vi "ADV Results Initiate.vi"(8 "error in":errorcluster, 10 "DAC ADV.lvclass":refnum<class "DAC ADV.lvclass">, 11 "Water Tunnel Results in":refnum<class "Water Tunnel Results.lvclass">) -> (0 "error out":errorcluster, 3 "Water Tunnel Results out":refnum<class "Water Tunnel Results.lvclass">)   [LabVIEW 2019, in "Results.lvlib" / "Water Tunnel Results.lvclass"]
uses:
  Water Tunnel Results.lvclass
  Water Tunnel Results.lvclass/Water Tunnel Results.ctl
  DAC/Water Tunnel/ADV/DAC ADV.lvclass
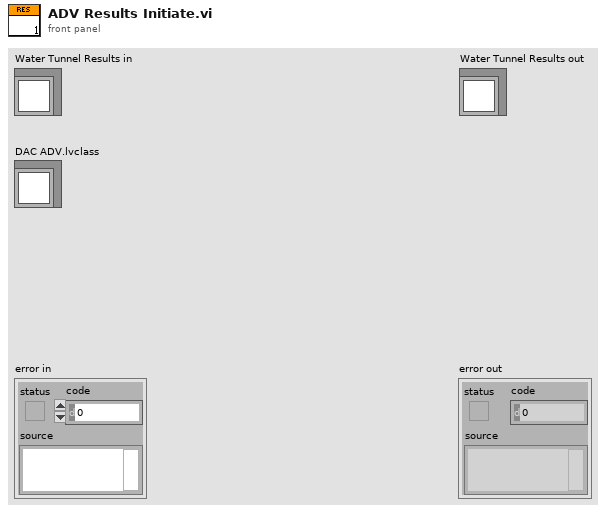
[diagram p1: front panel]
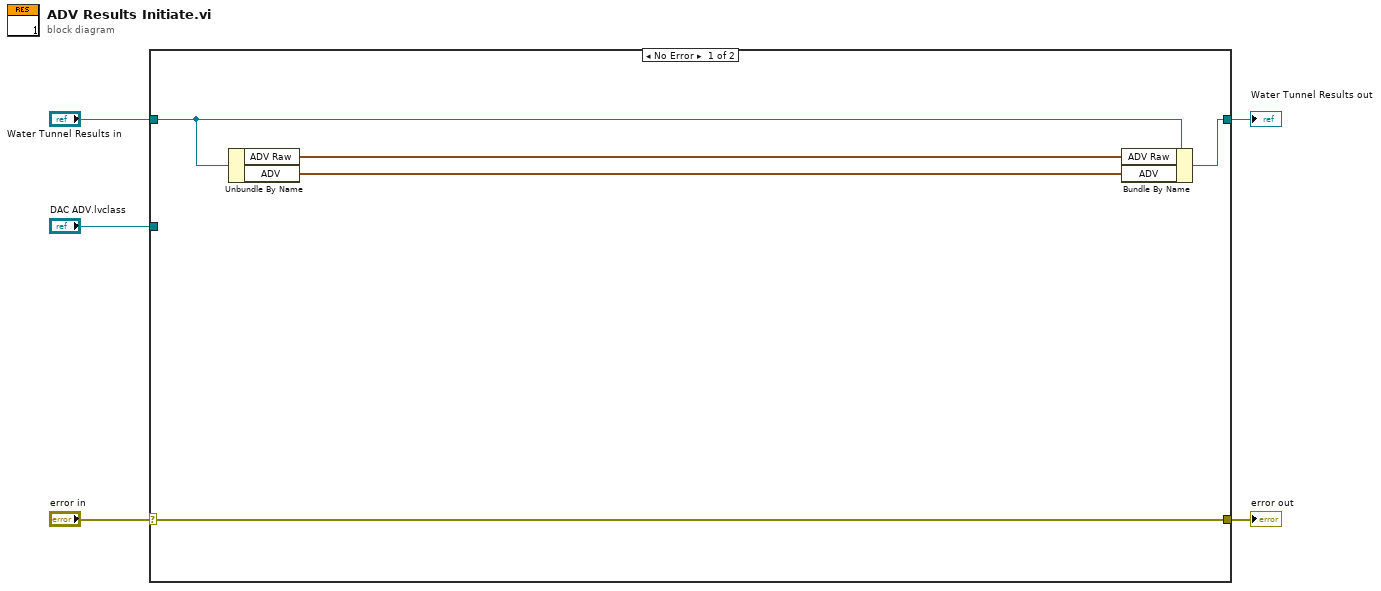
[diagram p0: block diagram]
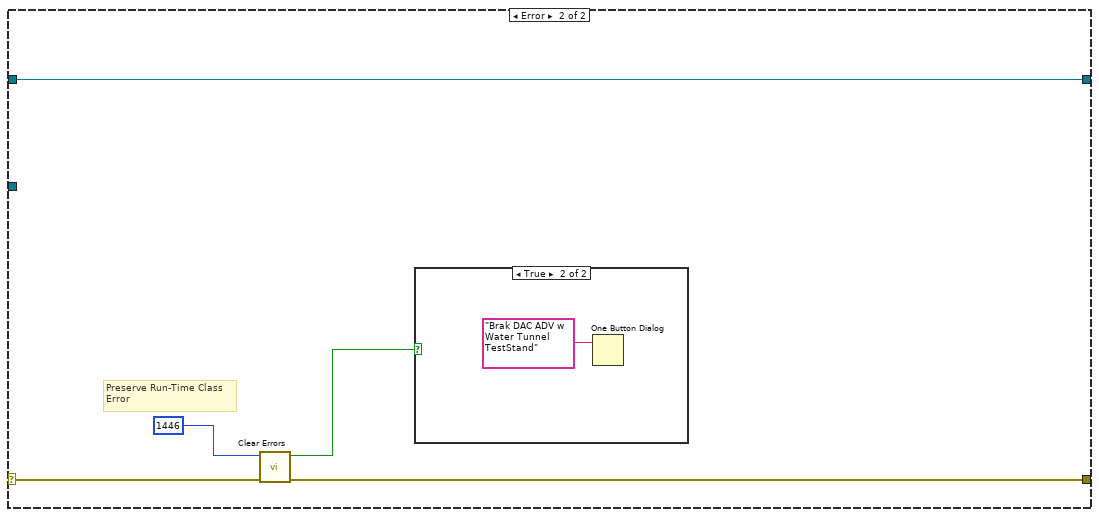
[diagram p2: hidden frame]
diagram:
  n1 = case shown="No Error" "error in" {
    selector: "error in" -> [w10 w14]
    tunnel: [w10 w13] -> w4
    tunnel: [w9 w15] -> w2
    tunnel: "Water Tunnel Results in" -> [w8 w15]
    tunnel: "DAC ADV.lvclass" -> [_ _]
    frame No Error {
      n2 = Unbundle By Name(w8) -> ("ADV Raw"=w7:waveform(dbl)[], "ADV"=w6:waveform(dbl)[])
      n3 = Bundle By Name(cluster=w8, "ADV Raw"=w7, "ADV"=w6) -> (w9:refnum<class "Water Tunnel Results.lvclass">)
    }
    frame Error {
      # "Preserve Run-Time Class\nError"
      n4 = call <vilib>:"Clear Errors.vi"("error in (no error)"=w14, "specific error code to clear (0: all)"=1446) -> ("error out"=w13:errorcluster, "specific error cleared?"=w11:bool)  [unwired: 4 in]
      n5 = case shown="True" w11 {
        frame False {
        }
        frame True {
          n6 = One Button Dialog(message="Brak DAC ADV w Water Tunnel TestStand") -> ()  [unwired: 1 in, 1 out]
        }
      }
    }
  }
  "error out" <- w4
  "Water Tunnel Results out" <- w2
